vi "Tree Up or Down Event.vi"(7 "Label":string, 10 "Up?":bool, 11 "GObject":refnum<vi>) -> ()   [LabVIEW 2021, in "Seq Edit Quick Drop.lvlib"]
uses:
  Seq Edit Quick Drop.lvlib
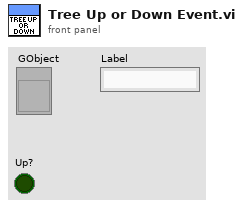
[diagram p1: front panel]
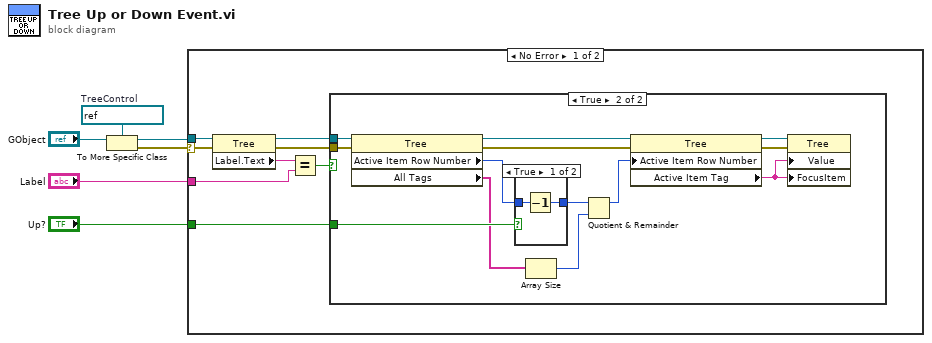
[diagram p0: block diagram]
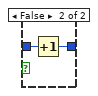
[diagram p3: hidden frame]
diagram:
  w2 = refnum<vi> refnum  # TreeControl
  n1 = To More Specific Class(target class=w2, reference="GObject") -> (specific class reference=w4:refnum<vi>, error out=w3:errorcluster)  [unwired: 1 in]
  n2 = case shown="No Error" w3 {
    selector: w3 -> [w12 _]
    tunnel: w4 -> [w13 _]
    tunnel: "Up?" -> [w9 _]
    tunnel: "Label" -> [w7 _]
    frame No Error {
      n3 = property class="Tree"(reference=w13, error in=w12) -> (reference out=w8:refnum<vi>, error out=w14:errorcluster, "Label.Text"=w11:string)
      n4 = Equal?(x=w11, y=w7) -> (x = y?=w10:bool)
      n5 = case shown="True" w10 {
        tunnel: w9 -> [_ w24]
        tunnel: w8 -> [_ w20]
        tunnel: w14 -> [_ w19]
        frame False {
        }
        frame True {
          n6 = property class="Tree"(reference=w20, error in=w19) -> (reference out=w26:refnum<vi>, error out=w18:errorcluster, "Active Item Row Number"=w27:i32, "All Tags"=w16:string[])
          n7 = case shown="True" w24 {
            tunnel: w27 -> [w29 w31]
            tunnel: [w28 w30] -> w25
            frame True {
              n8 = Decrement(x=w29) -> (x-1=w28:i32)
            }
            frame False {
              n9 = Increment(x=w31) -> (x+1=w30:i32)
            }
          }
          n10 = Array Size(array=w16) -> (size(s)=w15:i32)
          n11 = Quotient & Remainder(x=w25, y=w15) -> (x-y*floor(x/y)=w23:i32)  [unwired: 1 out]
          n12 = property class="Tree"(reference=w26, error in=w18, "Active Item Row Number"=w23) -> (reference out=w22:refnum<vi>, error out=w17:errorcluster, "Active Item Tag"=w21:string)
          n13 = property class="Tree"(reference=w22, error in=w17, "Value"=w21, "FocusItem"=w21) -> ()  [unwired: 2 out]
        }
      }
    }
    frame Error {
    }
  }
